vi "AVG.vi"(0 "System no.":i32=1 min=1 max=4 step=1, 3 "Averaging time":i16=1 min=0 max=20 step=1, 5 "error in":errorcluster) -> (14 "Controller error":bool, 19 "error out":errorcluster)   [LabVIEW 2020]
doc: "Sets averaging time to use for measurements. Controller error is TRUE if selected system reports an error code which is not 0.\n\nE-516: When making settings with AVG, they are automatically saved to flash ROM together with the current settings for the parameters listed below, and they become the new power-on defaults: \ncommunication interface, enabled channels and display format, drift compensation mode (DCO), velocity control mode (VCO) and velocity (VEL), offset and gain for position and output voltage display, mode and tolerance for on-target reading (SPA), position limits (PLM, NLM), voltage limits (VMA, VMI), macros and default macro setting.\nIf current parameter values are incorrect, the system may malfunction. Be sure that you have the correct parameter settings before using AVG.\n\nE-816: Averaging time (factor) can be 1, 2, 4, 8, 16, 32 or 64. This command cannot be issued to a slave\n\nE-761: Averaging (oversampling) time (factor) can be 4, 8, 16, 32, 64 or 128. The \"Sensor sampling time\" and \"Servo update time\" parameters are influenced by AVG. Use WPA.vi to save the values."
panel:
  # "Set averaging time to use for measurements."
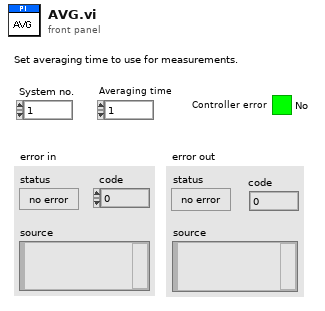
[diagram p1: front panel]
types:
  T1 = enum16{"Disable error check", "Force error check", "Use global settings"}
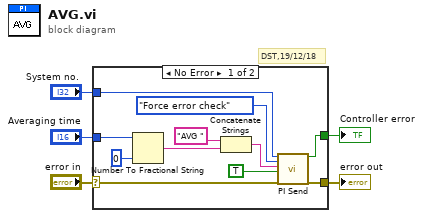
[diagram p0: block diagram]
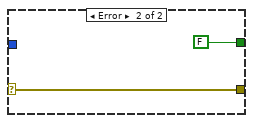
[diagram p2: hidden frame]
diagram:
  # "DST,19/12/18"
  n1 = case shown="No Error" "error in" {
    selector: "error in" -> [w9 w18]
    tunnel: [w8 w18] -> w5
    tunnel: "Averaging time" -> [w15 _]
    tunnel: "System no." -> [w11 _]
    tunnel: [w7 FALSE ("Controller error")] -> w2
    frame No Error {
      n2 = Number To Fractional String(number=w15, precision (6)=i16 0) -> (F-format string=w14:string)  [unwired: 2 out]
      n3 = Concatenate Strings("AVG ", w14) -> (w10:string)
      n4 = call "PI Send.vi"("System no."=w11, "Error check settings"=T1."Force error check", "String to send"=w10, "Attach termination char.?"=TRUE ("Attach Linefeed?"), "error in"=w9) -> ("Controller error"=w7:bool, "error out"=w8:errorcluster)  [unwired: 1 in, 12 out]
    }
    frame Error {
    }
  }
  "error out" <- w5
  "Controller error" <- w2
